vi "Read Counter Driven Output Module.vi"   [LabVIEW 2020, in "Scan Engine Scripting.lvlib"]
doc: "Returns the channel settings of a counter driven output module that can be edited and then used to create a new module instance to set into a slot."
uses:
  Scan Engine Scripting.lvlib
  Modules/NI 9475/NI 9475.lvclass
  Modules/NI 9474/NI 9474.lvclass
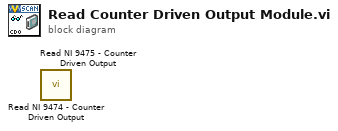
[diagram p0: block diagram]
diagram:
  n1 = call "Read NI 9474 - Counter Driven Output.vi"() -> ()  [unwired: 8 in, 4 out]
  n2 = call "Read NI 9475 - Counter Driven Output.vi"() -> ()  [unwired: 8 in, 4 out]
